vi "AddLayer toObstacle.vi"(6 "Intensity":dbl, 7 "Layer #":i32=1, 8 "map in":dbl[][](array[numeric]), 9 "y":i32, 10 "x":i32) -> (0 "map Out":dbl[][](array[numeric]), 1 "y out":i32, 2 "x out":i32)   [LabVIEW 2011]
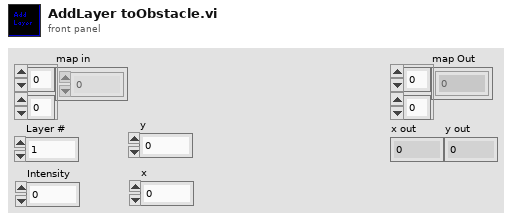
[diagram p1: front panel]
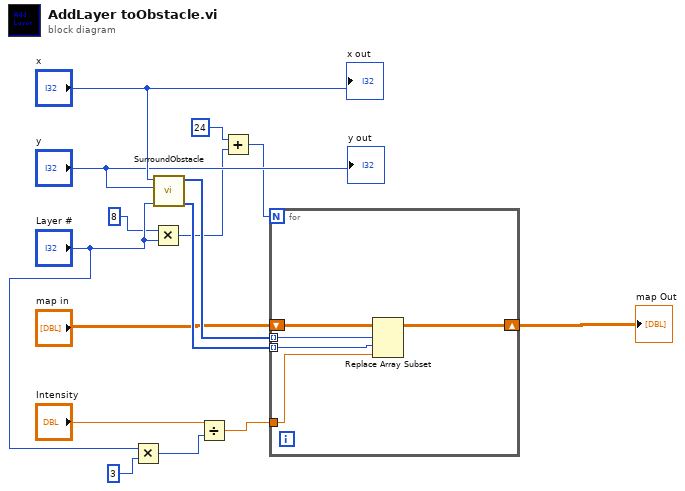
[diagram p0: block diagram]
diagram:
  n1 = Multiply(x="Layer #", y=3) -> (x*y=w7:i32)
  n2 = Multiply(x=8, y="Layer #") -> (x*y=w2:i32)
  n3 = call "SurroundObstacle.vi"("outside layer +1"="Layer #", "y"="y", "x"="x") -> ("y array"=w13:i32[], "x array"=w14:i32[])  [unwired: 7 in]
  n4 = Divide(x="Intensity", y=w7) -> (x/y=w15:dbl)
  n5 = Add(x=24, y=w2) -> (x+y=w1:i32)
  n6 = for {
    N: w1 -> [_]
    shift-right: [w20] -> w11
    shift-left: "map in" -> [w19]
    tunnel: w15 -> [w16]
    tunnel: w14 -> [w18] mode=indexing
    tunnel: w13 -> [w17] mode=indexing
    n7 = Replace Array Subset(array=w19, new element=w16, index (row)=w18, index (col)=w17) -> (w20:dbl[][])
  }
  "map Out" <- w11
  "x out" <- "x"
  "y out" <- "y"
